vi "SwitchPreCheck.vi"(9 "Max Dist":dbl=15.0 format="%#_13g", 10 "file path":path=path "D:/Minecraft/mmc-stable-win32/MultiMC/instances/TRAINS 3-/.minecraft/saves/trains/opencomputers/442cd0d6-e139-46e7-881b-600456d36bc7/home", 11 "All Lines in":T1) -> (1 "Changed?":bool, 3 "All Lines out":T1)   [LabVIEW 2014, in "Map Data.lvlib"]
uses:
  Map Data.lvlib
  All-Lines.ctl
  LineCluster.ctl
  LineConnection.ctl
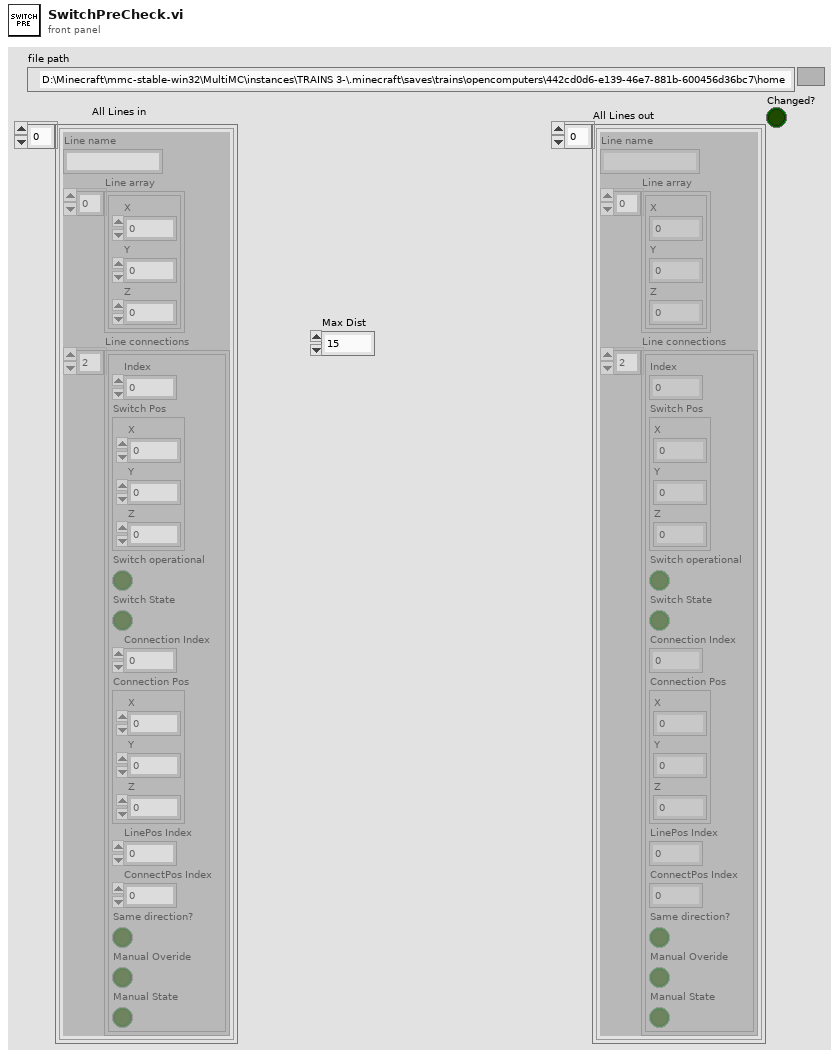
[diagram p1: front panel]
types:
  T1 = typedef "Map Data.lvlib/All-Lines.ctl" = T2[]
  T2 = typedef "Map Data.lvlib/LineCluster.ctl" = cluster{"Line name":string, "Line array":cluster{"X":dbl, "Y":dbl, "Z":dbl}[], "Line connections":T3[]}
  T3 = typedef "Map Data.lvlib/LineConnection.ctl" = cluster{"Index":i32, "Switch Pos":cluster{"X":dbl, "Y":dbl, "Z":dbl}, "Switch operational":bool, "Switch State":bool, "Connection Index":i32, "Connection Pos":cluster{"X":dbl, "Y":dbl, "Z":dbl}, "LinePos Index":i32, "ConnectPos Index":i32, "Same direction?":bool, "Manual Overide":bool, "Manual State":bool}
  T4 = enum16{"open", "replace", "create", "open or create", "replace or create", "replace or create with confirmation"}
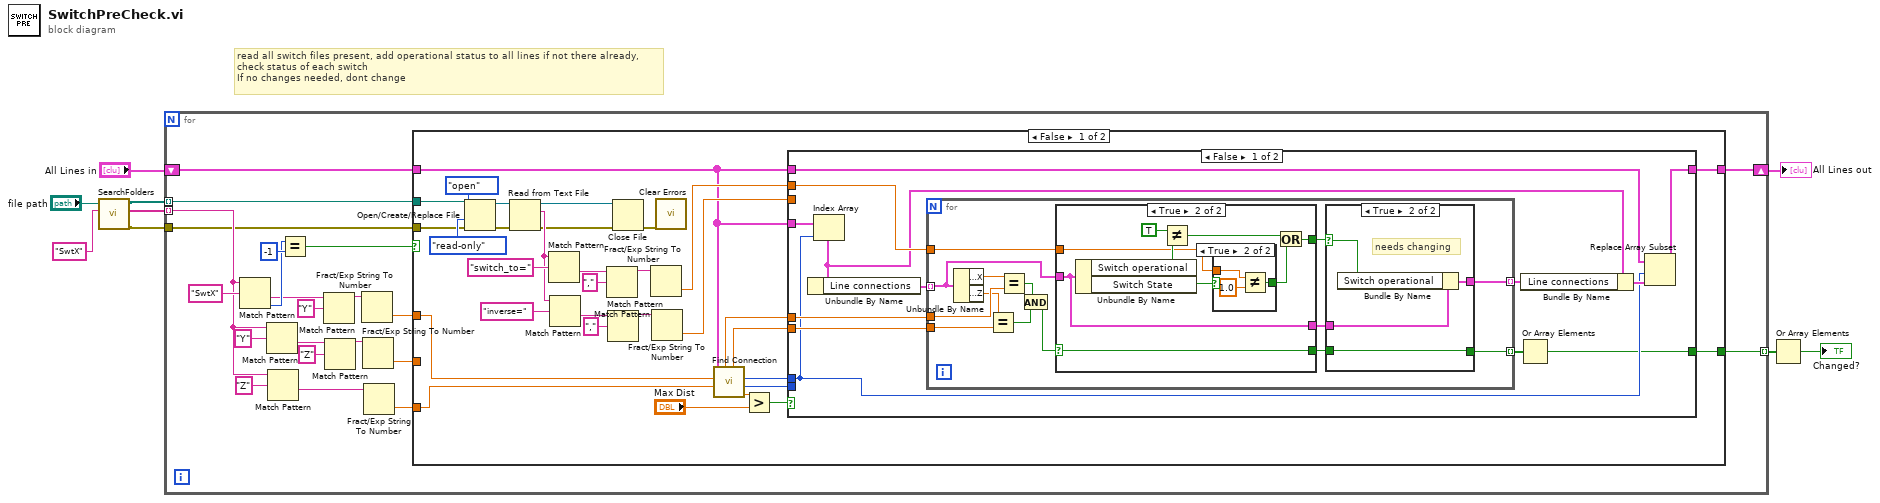
[diagram p0: block diagram]
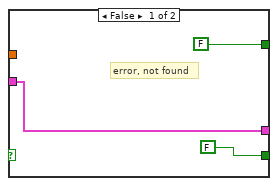
[diagram p3: hidden frame]
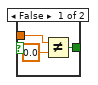
[diagram p4: hidden frame]
diagram:
  # "read all switch files present, add operational status to all lines if not there already,\ncheck status of each switch\nIf no changes needed, dont change"
  n1 = call "SearchFolders.vi"("regular expression"="SwtX", "file path"="file path") -> ("error out"=w4:errorcluster, "String Array"=w5:string[], "Path Array"=w6:path[])  [unwired: 6 in, 1 out]
  n2 = for {
    tunnel: w6 -> [w11] mode=indexing
    tunnel: w5 -> [w15] mode=indexing
    tunnel: w4 -> [w14]
    shift-right: [w12] -> w8
    shift-left: "All Lines in" -> [w13]
    tunnel: [w10] -> w2 mode=indexing
    n3 = Match Pattern(string=w15, regular expression="SwtX") -> (after substring=w20:string, offset past match=w30:i32)  [unwired: 1 in, 2 out]
    n4 = Match Pattern(string=w15, regular expression="Y" ("format string")) -> (after substring=w24:string)  [unwired: 1 in, 3 out]
    n5 = Match Pattern(string=w15, regular expression="Z" ("format string")) -> (after substring=w28:string)  [unwired: 1 in, 3 out]
    n6 = Equal?(x=w30, y=-1) -> (x = y?=w19:bool)
    n7 = Match Pattern(string=w20, regular expression="Y") -> (before substring=w21:string)  [unwired: 1 in, 3 out]
    n8 = Match Pattern(string=w24, regular expression="Z") -> (before substring=w26:string)  [unwired: 1 in, 3 out]
    n9 = Fract/Exp String To Number(string=w21) -> (number=w18:dbl)  [unwired: 3 in, 1 out]
    n10 = Fract/Exp String To Number(string=w26) -> (number=w17:dbl)  [unwired: 3 in, 1 out]
    n11 = Fract/Exp String To Number(string=w28) -> (number=w16:dbl)  [unwired: 3 in, 1 out]
    n12 = case shown="False" w19 {
      tunnel: w18 -> [w48 _]
      tunnel: w17 -> [_ _]
      tunnel: w16 -> [w47 _]
      tunnel: w14 -> [w61 _]
      tunnel: w13 -> [w37 w116]
      tunnel: [w36 w116] -> w12
      tunnel: w11 -> [w33 _]
      tunnel: [w32 _] -> w10
      frame False {
        n13 = Open/Create/Replace File(file path (use dialog)=w33, error in=w61, operation (0:open)=T4."open", access (0:read/write)=enum16{"read/write", "read-only", "write-only"}."read-only") -> (refnum out=w59:refnum<file>, error out=w60:errorcluster)  [unwired: 2 in, 1 out]
        n14 = Read from Text File(file (use dialog)=w59, error in=w60) -> (refnum out=w35:refnum<file>, text=w50:string, error out=w34:errorcluster)  [unwired: 2 in, 1 out]
        n15 = Match Pattern(string=w50, regular expression="switch_to=" ("format string")) -> (after substring=w49:string)  [unwired: 1 in, 3 out]
        n16 = Match Pattern(string=w50, regular expression="inverse=" ("format string")) -> (after substring=w55:string)  [unwired: 1 in, 3 out]
        n17 = Match Pattern(string=w49, regular expression=",") -> (before substring=w51:string)  [unwired: 1 in, 3 out]
        n18 = Match Pattern(string=w55, regular expression=",") -> (before substring=w57:string)  [unwired: 1 in, 3 out]
        n19 = Close File(refnum=w35, error in=w34) -> (error out=w58:errorcluster)  [unwired: 1 out]
        n20 = Fract/Exp String To Number(string=w51) -> (number=w39:dbl)  [unwired: 3 in, 1 out]
        n21 = Fract/Exp String To Number(string=w57) -> (number=w38:dbl)  [unwired: 3 in, 1 out]
        n22 = call <vilib>:"Clear Errors.vi"("error in (no error)"=w58) -> ()  [unwired: 5 in, 2 out]
        n23 = call "Find Connection.vi"("Z"=w47, "X"=w48, "All Lines"=w37) -> ("Distance to nearest"=w46:dbl, "Index on Line"=w43:i32, "Nearest Line"=w42:i32, "Z Coonnection"=w41:dbl, "X Connection"=w40:dbl)  [unwired: 2 in, 2 out]
        n24 = Greater?(x=w46, y="Max Dist") -> (0:w45:bool)
        n25 = case shown="False" w45 {
          tunnel: w43 -> [_ _]
          tunnel: w42 -> [w66 _]
          tunnel: w37 -> [w76 _]
          tunnel: w41 -> [w73 _]
          tunnel: w40 -> [w74 _]
          tunnel: w39 -> [w72 _]
          tunnel: w38 -> [_ _]
          tunnel: w37 -> [w68 w115]
          tunnel: [w65 w115] -> w36
          tunnel: [w64 _] -> w32
          frame False {
            n26 = Index Array(array=w76, index=w66) -> (element=w70:T2)
            n27 = Unbundle By Name(w70) -> ("Line connections"=w75:T3[])
            n28 = for {
              tunnel: w75 -> [w84] mode=indexing
              tunnel: w74 -> [w89]
              tunnel: w73 -> [w87]
              tunnel: w72 -> [w83]
              tunnel: [w78] -> w69 mode=indexing
              tunnel: [w77] -> w71 mode=indexing
              n29 = Unbundle By Name(w84) -> ("Switch Pos.X"=w90:dbl, "Switch Pos.Z"=w88:dbl)
              n30 = Equal?(x=w88, y=w87) -> (x = y?=w85:bool)
              n31 = Equal?(x=w90, y=w89) -> (x = y?=w86:bool)
              n32 = And(x=w86, y=w85) -> (x .and. y?=w79:bool)
              n33 = case shown="True" w79 {
                selector: w79 -> [_ w101]
                tunnel: w84 -> [w97 w100]
                tunnel: w83 -> [_ w103]
                tunnel: [FALSE w102] -> w82
                tunnel: [FALSE w101] -> w80
                tunnel: [w97 w100] -> w81
                frame False {
                  # "error, not found"
                }
                frame True {
                  n34 = Unbundle By Name(w100) -> ("Switch operational"=w108:bool, "Switch State"=w106:bool)
                  n35 = Not Equal?(x=TRUE, y=w108) -> (x != y?=w105:bool)
                  n36 = case shown="True" w106 {
                    tunnel: w103 -> [w110 w114]
                    tunnel: [w109 w112] -> w104
                    frame False {
                      n37 = Not Equal?(x=w110, y=0.0) -> (x != y?=w109:bool)
                    }
                    frame True {
                      n38 = Not Equal?(x=w114, y=1.0) -> (x != y?=w112:bool)
                    }
                  }
                  n39 = Or(x=w105, y=w104) -> (x .or. y?=w102:bool)
                }
              }
              n40 = case shown="True" w82 {
                selector: w82 -> [_ w95]
                tunnel: w81 -> [w92 w96]
                tunnel: [w92 w94] -> w78
                tunnel: [w91 w93] -> w77
                tunnel: w80 -> [w91 w93]
                frame False {
                }
                frame True {
                  # "needs changing"
                  n41 = Bundle By Name(cluster=w96, "Switch operational"=w95) -> (w94:T3)
                }
              }
            }
            n42 = Or Array Elements(Boolean array=w71) -> (logical OR=w64:bool)
            n43 = Bundle By Name(cluster=w70, "Line connections"=w69) -> (w67:T2)
            n44 = Replace Array Subset(array=w68, new element=w67, index=w66) -> (w65:T1)
          }
          frame True {
            # "error\nswitch file found\nno switches within the distance"
          }
        }
      }
      frame True {
      }
    }
  }
  "All Lines out" <- w8
  n45 = Or Array Elements(Boolean array=w2) -> (logical OR=→"Changed?":bool)
